vi "REQ Update User Details.vi"(8 "error in":errorcluster, 10 "Update Credential":T1) -> (0 "error out":errorcluster)   [LabVIEW 2016, in "Database.lvlib"]
doc: "_____\nCreated using DQMH Event Scripter 7.0.0.1280."
uses:
  Database.lvlib
  REQ Update User Details Argument--cluster.ctl
  Class/DB/Update Credential.ctl
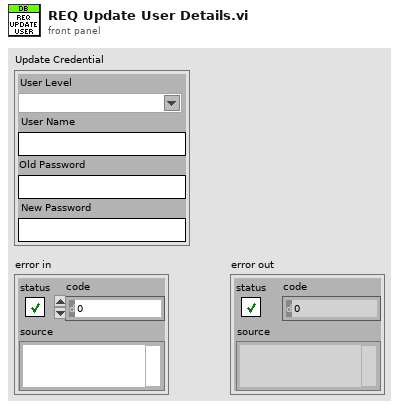
[diagram p1: front panel]
types:
  T1 = typedef "Database.lvlib/Update Credential.ctl" = cluster{"User Level":string, "User Name":string, "Old Password":string, "New Password":string}
  T2 = typedef "Database.lvlib/REQ Update User Details Argument--cluster.ctl" = cluster{"Update Credential":T1}
  T3 = typedef "Database.lvlib/Request Events--cluster.ctl" = cluster{"Stop Module":refnum<user-event>, "Show Panel":refnum<user-event>, "Hide Panel":refnum<user-event>, "Get Module Execution Status":refnum<user-event>, "Show Diagram":refnum<user-event>, "REQ Add User":refnum<user-event>, "REQ Check Credential":refnum<user-event>, "REQ Delete User":refnum<user-event>, "REQ Update User Details":refnum<user-event>, "REQ List Table":refnum<user-event>, "REQ Delete Table Data":refnum<user-event>, "REQ Save DB Record Data":refnum<user-event>, "REQ Save Test Data":refnum<user-event>, "REQ Load Test Data":refnum<user-event>, "REQ Get Username":refnum<user-event>, "REQ Close DB Ref":refnum<user-event>, "REQ Retry DB":refnum<user-event>, "REQ DB Setup":refnum<user-event>, "REQ Write Test Info":refnum<user-event>, "REQ Fetch Coulmn Name":refnum<user-event>}
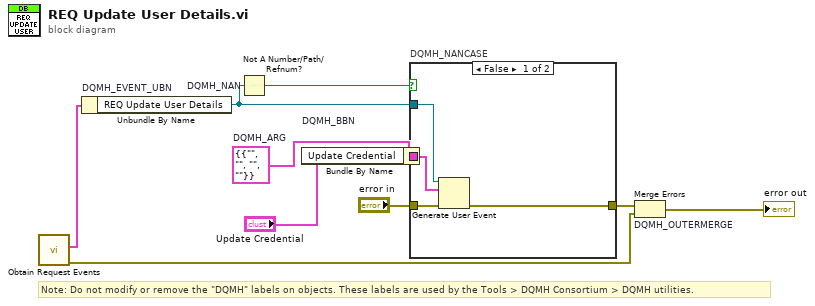
[diagram p0: block diagram]
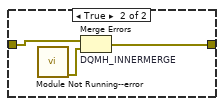
[diagram p2: hidden frame]
diagram:
  w4 = T2 {"Update Credential"={"User Level"="", "User Name"="", "Old Password"="", "New Password"=""}}  # DQMH_ARG
  # "Note: Do not modify or remove the \"DQMH\" labels on objects. These labels are used by the Tools > DQMH Consortium > DQMH utilities."
  n1 = call "Obtain Request Events.vi"() -> ("error out"=w2:errorcluster, "Database Request Events"=w1:T3)  [unwired: 10 in]
  n2 = Unbundle By Name "DQMH_EVENT_UBN"(w1) -> ("REQ Update User Details"=w6:refnum<user-event>)
  n3 = Not A Number/Path/Refnum? "DQMH_NAN"(number/path/refnum=w6) -> (NaN/Path/Refnum?=w7:bool)
  n4 = Bundle By Name "DQMH_BBN"(cluster=w4, "Update Credential"="Update Credential") -> (w8:T2)
  n5 = case "DQMH_NANCASE" shown="False" w7 {
    tunnel: "error in" -> [w14 w17]
    tunnel: [w13 w16] -> w5
    tunnel: w6 -> [w12 _]
    tunnel: w8 -> [w11 _]
    frame False {
      n6 = Generate User Event(user event=w12, event data cluster=w11, error in=w14) -> (error out=w13:errorcluster)  [unwired: 1 in, 1 out]
    }
    frame True {
      n7 = call "Module Not Running--error.vi"() -> ("error out"=w15:errorcluster)  [unwired: 11 in]
      n8 = Merge Errors "DQMH_INNERMERGE"(w17, w15) -> (w16:errorcluster)
    }
  }
  n9 = Merge Errors "DQMH_OUTERMERGE"(w5, w2) -> (→"error out":errorcluster)
